vi "Split Boolean Array into Integer Array.vi"(10 "Array":bool[](array[boolean])) -> (2 "appended array":u64[](array[numeric]) format="%064b")   [LabVIEW 2015]
panel:
  out "First subarray":bool[](array[boolean])
  out "Second subarray":bool[](array[boolean])
  out "Third subarray":bool[](array[boolean])
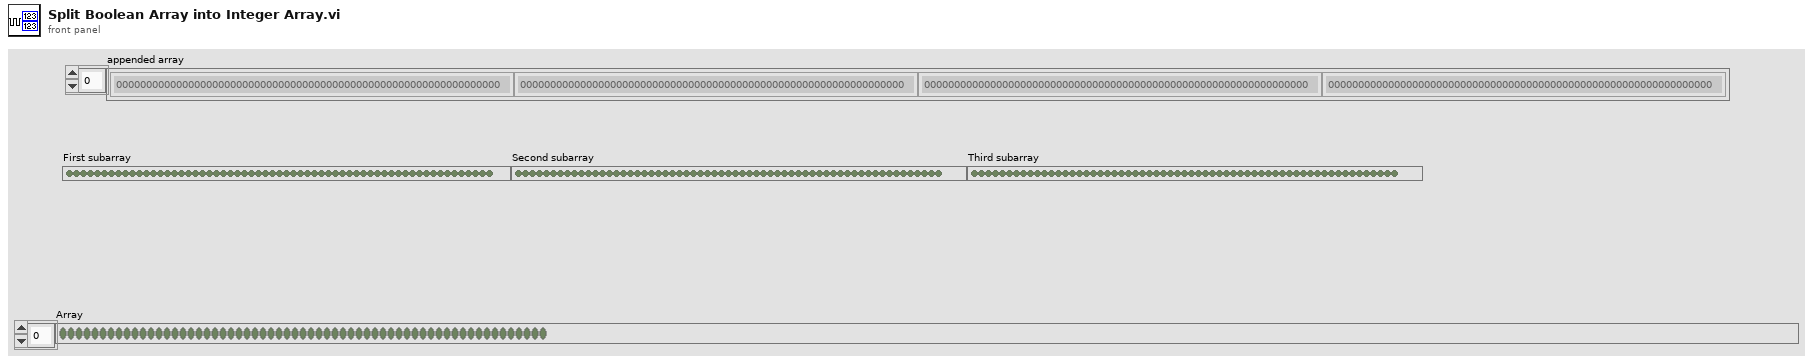
[diagram p1: front panel]
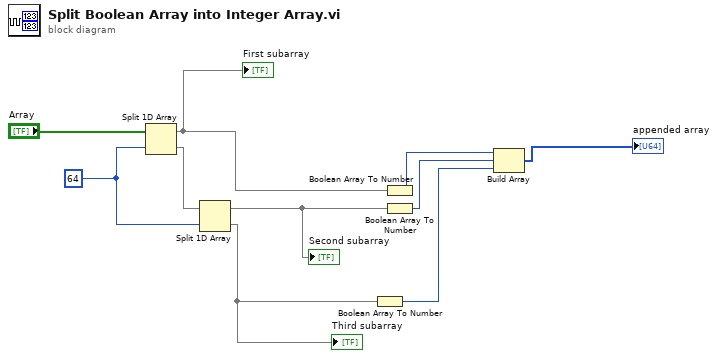
[diagram p0: block diagram]
diagram:
  w9 = 64 ("index")
  n1 = Split 1D Array(array="Array", index=w9) -> (first subarray=w5:bool[], second subarray=w8:bool[])
  "First subarray" <- w5
  n2 = Split 1D Array(array=w8, index=w9) -> (first subarray=w3:bool[], second subarray=w6:bool[])
  "Third subarray" <- w6
  "Second subarray" <- w3
  n3 = Boolean Array To Number(Boolean array=w6) -> (number=w7:u64)
  n4 = Boolean Array To Number(Boolean array=w5) -> (number=w1:u64)
  n5 = Boolean Array To Number(Boolean array=w3) -> (number=w2:u64)
  n6 = Build Array(w1, w2, w7) -> (→"appended array":u64[])
